vi "writeToXML.vi"(8 "error in (no error)":errorcluster, 10 "ClassLabel":string, 11 "ScienceTargetOffset in":refnum<class "ScienceTargetOffset.lvclass">) -> (0 "error out":errorcluster, 2 "XML out":string, 3 "ScienceTargetOffset out":refnum<class "ScienceTargetOffset.lvclass">)   [LabVIEW 2022 SP3, in "TCSDataDefinitions.lvlib" / "TCSCommand.lvlib" / "OffsetCommands.lvlib" / "ScienceTargetOffset.lvclass"]
uses:
  ScienceTargetOffset.lvclass
  Offset/Offset.lvclass
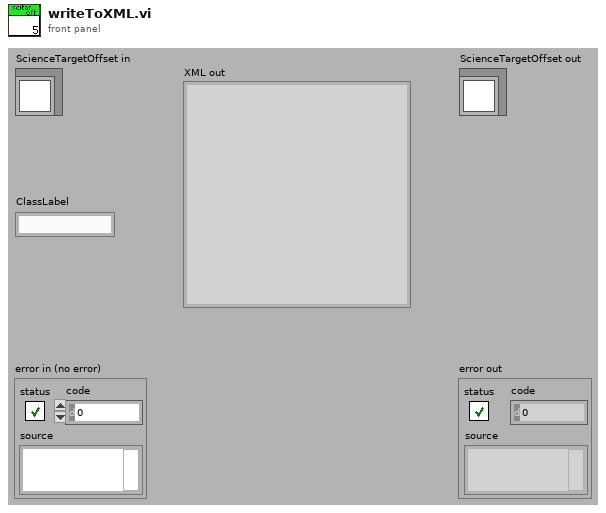
[diagram p1: front panel]
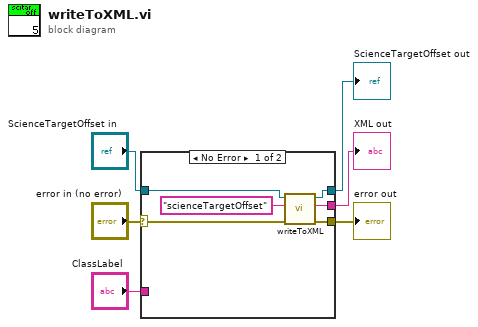
[diagram p0: block diagram]
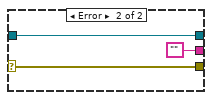
[diagram p2: hidden frame]
diagram:
  n1 = case shown="No Error" "error in (no error)" {
    selector: "error in (no error)" -> [w9 w15]
    tunnel: [w8 w15] -> w5
    tunnel: [w11 w14] -> w3
    tunnel: "ScienceTargetOffset in" -> [w12 w14]
    tunnel: [w10 ""] -> w2
    tunnel: "ClassLabel" -> [_ _]
    frame No Error {
      n2 = call-parent "writeToXML.vi"("error in (no error)"=w9, "ClassLabel"="scienceTargetOffset", "Offset in"=w12) -> ("error out"=w8:errorcluster, "XML out"=w10:string, "Offset out"=w11:refnum<class "ScienceTargetOffset.lvclass">)  [unwired: 6 in]
    }
    frame Error {
    }
  }
  "error out" <- w5
  "ScienceTargetOffset out" <- w3
  "XML out" <- w2
